vi "Play Timing Module.vi"(7 "Commands":T2=enum."Initialize", 8 "error in":errorcluster, 9 "Rotation Resolution":dbl=20.0, 10 "Facets To move":T1[](array[typedef]), 11 "Axis":cluster{"X":sgl, "Y":sgl, "Z":sgl}) -> (0 "error out":errorcluster)   [LabVIEW 2019]
uses:
  Play timing module commands.ctl
  Rubix Array data type.ctl
  <vilib>/Platform/TimedLoop/XDataNode/timing_clust.ctl
  <vilib>/Platform/TimedLoop/XDataNode/nitl_modes.ctl
  <vilib>/Platform/TimedLoop/XDataNode/wakeup.ctl
  Scene Commands.ctl
  <vilib>/Platform/TimedLoop/scheduler/LVUserAPI/_suppVIs/Create_1kHz_TSource.vi
  <vilib>/Platform/TimedLoop/XDataNode/XDataNode.xnode
  <vilib>/Platform/TimedLoop/XDataNode/XDNodeRunTimeDep.lvlib
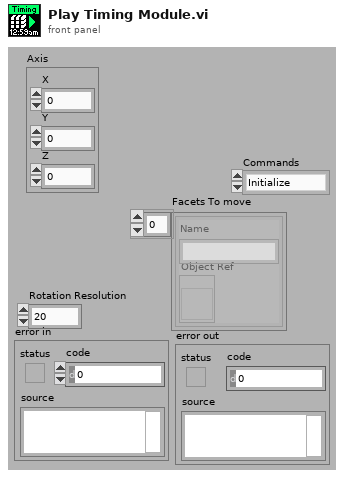
[diagram p1: front panel]
types:
  T1 = typedef "Rubix Array data type.ctl" = cluster{"Object Ref":refnum<vi>, "Name":string}
  T2 = typedef "Play timing module commands.ctl" = enum16{"Clean up", "Initialize", "Run"}
  T3 = typedef "Scene Commands.ctl" = enum16{"Init", "Set Rubix Text Array", "Get Rubix Ref Array", "Generate Rubix Array", "Get Rubix Array", "Show Render Window", "Go To Face", "Rotate", "Update Scene", "Clear Rubix"}
  T4 = typedef "XDNodeRunTimeDep.lvlib/timing_clust.ctl" = cluster{"Expected End [f-1]":u64, "Actual End [f-1]":u64, "Finished Late? [f-1]":bool, "Expected End [i-1]":u64, "Actual End [i-1]":u64, "Finished Late? [i-1]":bool, "Expected Start [i]":u64, "Actual Start [i]":u64, "Expected Start [f]":u64, "Actual Start [f]":u64, "Source Name":string, "Structure Name":string, "Period":i64, "Deadline":i64, "Offset":i64, "Start":i64, "Priority":i32, "Timeout":i32, "Mode":T5, "Wakeup Reason":T6, "Error":errorcluster, "Source Type":string, "Secondary Source Type":string, "Global End Time":u64, "Global Start Time":u64, "Frame Duration":u64, "Iteration Duration":u64, "Assigned CPU":i32, "I/O Scan Engine Mode":u32}
  T5 = typedef "XDNodeRunTimeDep.lvlib/nitl_modes.ctl" = enum32{"No Change", "Process missed periods, maintain original phase", "Discard missed periods, maintain original phase", "Process missed periods, ignore original phase", "Discard missed periods, ignore original phase"}
  T6 = typedef "XDNodeRunTimeDep.lvlib/wakeup.ctl" = enum32{"Normal", "Aborted", "Asynchronous wakeup", "Timing source error", "Timed loop error", "Timeout"}
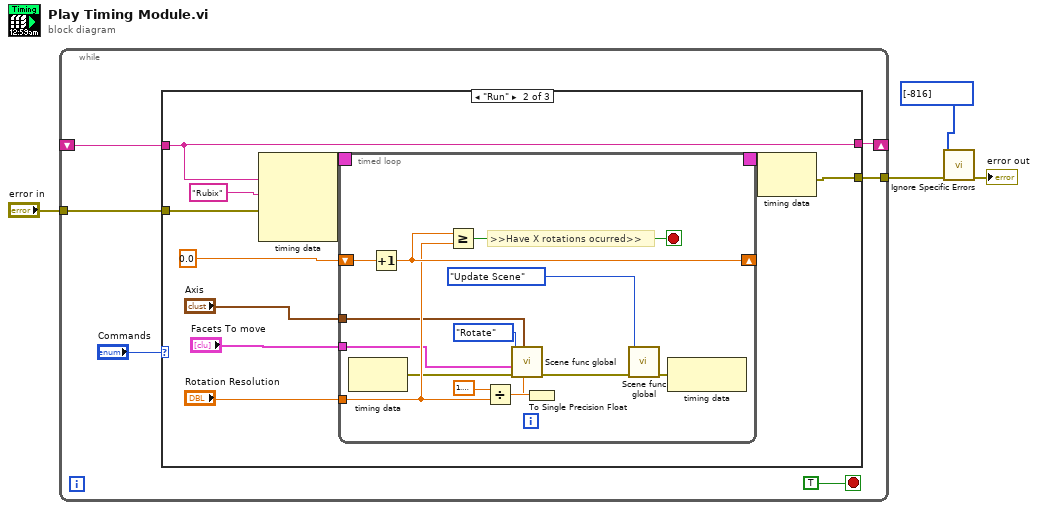
[diagram p0: block diagram]
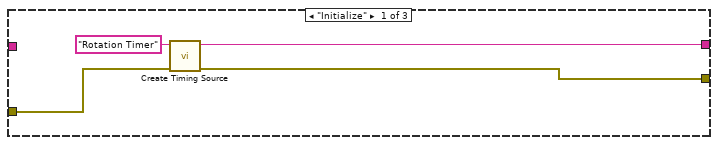
[diagram p2: hidden frame]
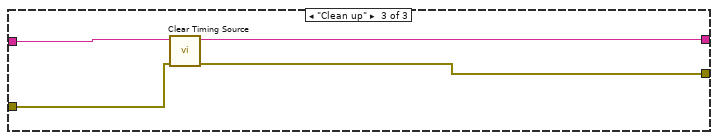
[diagram p3: hidden frame]
diagram:
  n1 = while {
    tunnel: "error in" -> [w5]
    tunnel: [w9] -> w1
    shift-right: [w7] -> _
    shift-left: _ -> [w6]
    stop <- TRUE stop-if-true
    n2 = case shown="\"Run\"" "Commands" {
      tunnel: [w11 w16 w51] -> w9
      tunnel: [w14 w19 w53] -> w7
      tunnel: w6 -> [_ w19 w53]
      tunnel: w5 -> [w12 w17 w52]
      frame "Initialize" {
        n3 = call-poly <vilib>:"Create Timing Source.vi"("error in (no error)"=w12, "name (in)"="Rotation Timer") -> ("error out"=w11:errorcluster, "name (out)"=w14:string)  [unwired: 8 in]
      }
      frame "Run" {
        n4 = node-c288(w19, "Rubix" ("Name"), w17) -> (w24:T4)  [unwired: 1 in]
        n5 = timed-loop {
          timing: w24 -> [_]
          timing-out: [_] -> w23
          shift-right: [w35] -> _
          shift-left: 0.0 -> [w34]
          tunnel: "Rotation Resolution" -> [w33]
          tunnel: "Axis" -> [w30]
          tunnel: "Facets To move" -> [w28]
          stop <- w36 stop-if-true
          # ">>Have X rotations ocurred>>"
          n6 = node-c288() -> (w29:errorcluster)  [unwired: 1 in]
          n7 = Increment(x=w34) -> (x+1=w35:dbl)
          n8 = Greater Or Equal?(x=w35, y=w33) -> (x >= y?=w36:bool)
          n9 = Divide(x=1.5707963267948966, y=w33) -> (x/y=w37:dbl)
          n10 = To Single Precision Float(number=w37) -> (single precision float=w31:sgl)
          n11 = call "Scene func global.vi"("Angle"=w31, "Axis"=w30, "error in (no error)"=w29, "Facets To move"=w28, "Commands"=Scene_Commands."Rotate") -> ("error out"=w25:errorcluster)  [unwired: 5 in, 1 out]
          n12 = call "Scene func global.vi"("error in (no error)"=w25, "Commands"=Scene_Commands."Update Scene") -> ("error out"=w27:errorcluster)  [unwired: 8 in, 1 out]
          n13 = node-c288(w27) -> ()  [unwired: 1 out]
        }
        n14 = node-c288(w23) -> (w16:errorcluster)
      }
      frame "Clean up" {
        n15 = call <vilib>:"Clear Timing Source.vi"("error in (no error)"=w52, "name"=w53) -> ("error out"=w51:errorcluster)  [unwired: 8 in, 1 out]
      }
    }
  }
  n16 = call "Ignore Specific Errors.vi"("error in (no error)"=w1, "Array"=i32[] [-816]) -> ("error out"=→"error out":errorcluster)  [unwired: 8 in, 1 out]
